vi "Player Info.vi"(11 "Borg in":refnum<class "Borg.lvclass">) -> (1 "Victory Speech":string, 2 "Name":string, 3 "Borg out":refnum<class "Borg.lvclass">)   [LabVIEW 2015, in "Borg.lvclass"]
uses:
  Borg.lvclass
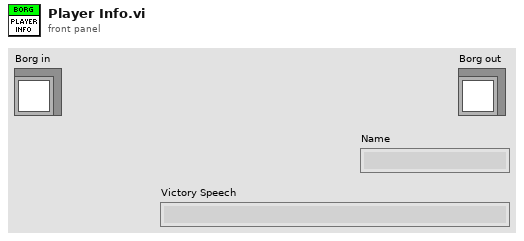
[diagram p1: front panel]
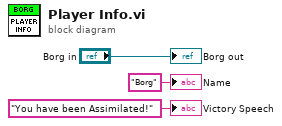
[diagram p0: block diagram]
diagram:
  "Borg out" <- "Borg in"
  "Name" <- "Borg" ("Name")
  "Victory Speech" <- "You have been Assimilated!" ("Victory Speech")
